vi "Read.vi"(4 "TypeMap in":refnum<class "TypeMap.lvclass">, 6 "commandTimeout":i32=-1, 7 "Explicit Where (first array element) [F]":bool, 8 "error in (no error)":errorcluster, 9 "Where":string[](array[string]), 10 "object in":refnum<class>, 11 "SqlMapper in":refnum<class "SqlMapper.lvclass">) -> (0 "error out":errorcluster, 1 "NotFound":bool, 2 "object out":refnum<class>, 3 "SqlMapper out":refnum<class "SqlMapper.lvclass">)   [LabVIEW 2020, in "ORM_API.lvlib"]
doc: "Get a single entity by ID."
uses:
  ORM_API.lvlib
  <vilib>/Viviota/shared/ORM.lvlibp/ORM/TypeMap/TypeMap.lvclass
  <vilib>/Viviota/shared/ORM.lvlibp/ORM/SqlMapper/SqlMapper.lvclass
  <userlib>/_OpenG.lib/lvdata/lvdata.llb/LVOOP Is Default Value__ogtk.vi
  <vilib>/Viviota/shared/ORM.lvlibp/ORM/TypeMap/Read TypeMap.vi
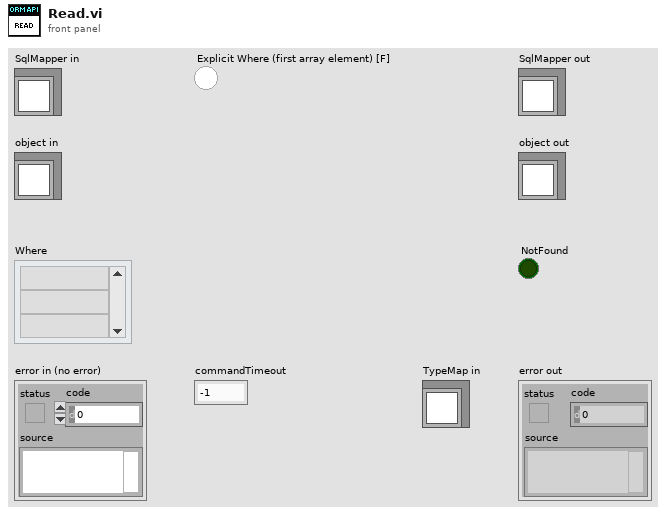
[diagram p1: front panel]
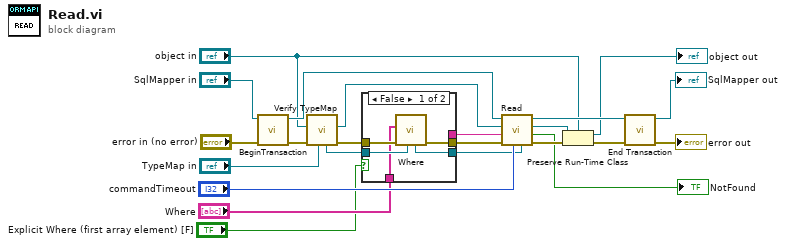
[diagram p0: block diagram]
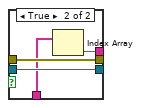
[diagram p2: hidden frame]
diagram:
  n1 = call-dynamic "BeginTransaction.vi"("error in (no error)"="error in (no error)", "SqlMapper in"="SqlMapper in") -> ("error out"=w21:errorcluster, "SqlMapper out"=w18:refnum<class "SqlMapper.lvclass">)  [unwired: 8 in]
  n2 = call "Verify TypeMap.vi"("TypeMap in"="TypeMap in", "error in (no error)"=w21, "Type in"="object in") -> ("error out"=w13:errorcluster, "Type out"=w14:refnum<class>, "TypeMap out"=w11:refnum<class "TypeMap.lvclass">)  [unwired: 6 in]
  n3 = case shown="False" "Explicit Where (first array element) [F]" {
    tunnel: w13 -> [w28 w31]
    tunnel: [w27 w31] -> w12
    tunnel: w11 -> [w26 w32]
    tunnel: [w25 w32] -> w10
    tunnel: "Where" -> [w24 w30]
    tunnel: [_ w29] -> w6
    frame False {
      n4 = call <vilib>:"Where.vi"("TypeMap in"=w26, "error in (no error)"=w28, "Where in"=w24) -> ("error out"=w27:errorcluster, "TypeMap out"=w25:refnum<class "TypeMap.lvclass">)  [unwired: 7 in]
    }
    frame True {
      n5 = Index Array(array=w30) -> (element=w29:string)  [unwired: 1 in]
    }
  }
  n6 = call-dynamic "Read.vi"("TypeMap in"=w10, "commandTimeout"="commandTimeout", "error in (no error)"=w12, "Where"=w6, "object in"=w14, "SqlMapper in"=w18) -> ("error out"=w9:errorcluster, "NotFound"=→"NotFound":bool, "Value"=w3:refnum<class>, "SqlMapper out"=w16:refnum<class "SqlMapper.lvclass">)  [unwired: 2 in]
  n7 = Preserve Run-Time Class(object in=w3, error in=w9, 2:"object in") -> (object out=→"object out":refnum<class>, error out=w4:errorcluster)
  n8 = call <vilib>:"End Transaction.vi"("error in (no error)"=w4, "SqlMapper in"=w16) -> ("error out"=→"error out":errorcluster, "SqlMapper out"=→"SqlMapper out":refnum<class "SqlMapper.lvclass">)  [unwired: 8 in]
